vi "Adjust for DST.vi"(9 "Adjust for DST? (T)":bool=TRUE, 10 "Timestamp":timestamp) -> (2 "Adjusted Timestamp":timestamp)   [LabVIEW 2013, in "DateTimeFormatter.lvclass"]
uses:
  DateTimeFormatter.lvclass
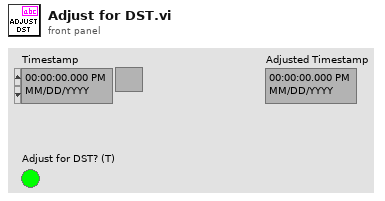
[diagram p1: front panel]
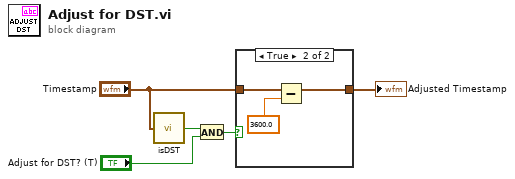
[diagram p0: block diagram]
diagram:
  n1 = call "isDST.vi"("timestamp (now)"="Timestamp") -> ("is DST?"=w5:bool)  [unwired: 8 in]
  n2 = And(x=w5, y="Adjust for DST? (T)") -> (x .and. y?=w4:bool)
  n3 = case shown="True" w4 {
    tunnel: [w6 w7] -> w3
    tunnel: "Timestamp" -> [w6 w9]
    frame False {
    }
    frame True {
      n4 = Subtract(x=w9, y=3600.0 ("x-y")) -> (x-y=w7:timestamp)
    }
  }
  "Adjusted Timestamp" <- w3
